vi "Cam Close (SubVI).vi"(8 "error in (no error)":errorcluster, 10 "Refnum in":T2, 11 "Refnum in":T1) -> (0 "error out":errorcluster)   [LabVIEW 2013]
uses:
  <vilib>/vision/Image Controls.llb/IMAQ Image.ctl
  <vilib>/userdefined/High Color/IMAQdx.ctl
  <vilib>/vision/driver/NI_Vision_Acquisition_Software.lvlib
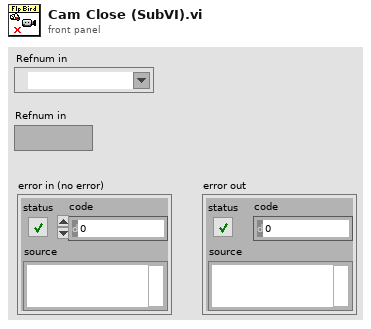
[diagram p1: front panel]
types:
  T1 = typedef "IMAQdx.ctl" = refnum<k21>
  T2 = typedef "IMAQ Image.ctl" = refnum<image>
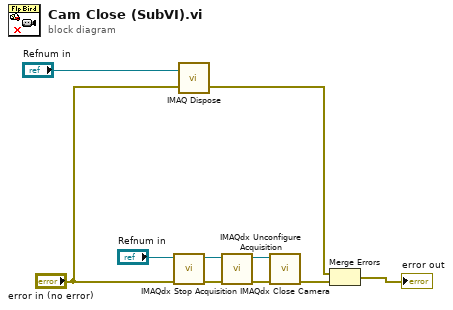
[diagram p0: block diagram]
diagram:
  n1 = call <vilib>:"IMAQdx Stop Acquisition.vi"("error in"="error in (no error)", "Session In"="Refnum in") -> ("error out"=w5:errorcluster, "Session Out"=w6:T1)  [unwired: 8 out]
  n2 = call "IMAQ Dispose"("Image"="Refnum in", "error in (no error)"="error in (no error)") -> ("error out"=w1:errorcluster)  [unwired: 4 in]
  n3 = call <vilib>:"IMAQdx Unconfigure Acquisition.vi"("error in"=w5, "Session In"=w6) -> ("error out"=w8:errorcluster, "Session Out"=w7:T1)  [unwired: 8 out]
  n4 = call <vilib>:"IMAQdx Close Camera.vi"("error in"=w8, "Session In"=w7) -> ("error out"=w4:errorcluster)  [unwired: 9 out]
  n5 = Merge Errors(w1, w4) -> (→"error out":errorcluster)
